vi "PZT frequency set.vi"(2 "error in (no error)":errorcluster caption="错误输入（无错误）", 3 "频率（Hz）":i32, 4 "VISA resource name":refnum<visa-resource-name> caption="VISA资源名称") -> (0 "错误输出":errorcluster, 1 "VISA资源名称输出":refnum<visa-resource-name>)   [LabVIEW 2019]
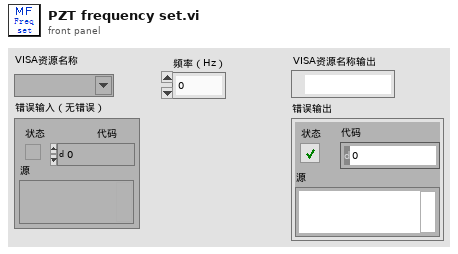
[diagram p1: front panel]
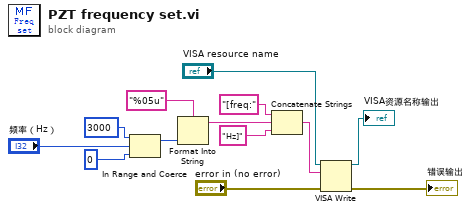
[diagram p0: block diagram]
diagram:
  n1 = In Range and Coerce(upper limit=3000 ("上限"), x="频率（Hz）", lower limit=0 ("下限")) -> (coerced(x)=w1:i32)  [unwired: 1 out]
  n2 = Format Into String(format string="%05u" ("格式字符串"), w1) -> (resulting string=w8:string)  [unwired: 2 in, 1 out]
  n3 = Concatenate Strings("[freq:" ("字符串"), w8, "Hz]" ("字符串")) -> (w5:string)
  n4 = VISA Write(VISA resource name="VISA resource name", write buffer=w5, error in (no error)="error in (no error)") -> (VISA resource name out=→"VISA资源名称输出":refnum<visa-resource-name>, error out=→"错误输出":errorcluster)  [unwired: 1 out]
